vi "Integrate_Gyro.vi"(10 "Dt":dbl, 11 "gyro[0]":sgl) -> (3 "Integrated Gyro":dbl)   [LabVIEW 2014]
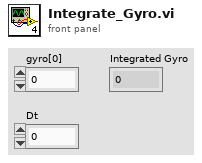
[diagram p1: front panel]
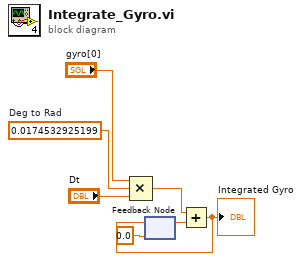
[diagram p0: block diagram]
diagram:
  w5 = 0.0174532925199  # Deg to Rad
  n1 = Compound Arithmetic op=MULTIPLY("gyro[0]", w5, "Dt") -> (w1:dbl)
  n2 = feedback #1(0.0) -> (w2:dbl)
  n3 = Add(x=w1, y=w2) -> (x+y=w7:dbl)
  "Integrated Gyro" <- w7
  n4 = feedback-in #1(w7) -> ()
